vi "sensor count.vi"(0 "sensor thr array":dbl[](array[numeric]), 1 "debounce time":dbl=0.25 format="%#_13g", 5 "capture y or no ?":bool, 7 "sensor data":dbl[](array[numeric]), 9 "counter input":dbl, 11 "counting role":T1(ring), 12 "error in":errorcluster, 13 "falling level thr":dbl=59000.0 format="%#_13g") -> (2 "machine pallet stop":bool, 3 "column count":bool, 4 "capture trigger":bool, 6 "sensor counter":bool, 8 "speed":dbl, 10 "counter out":dbl, 14 "pallet detect":bool, 15 "error out":errorcluster)   [LabVIEW 2019]
uses:
  <vilib>/measure/mamon.llb/Trigger Detection for 1 Channel.vi
  <vilib>/measure/NI_MAPro.lvlib
panel:
  out "coloumn read time 2":dbl caption="Elapsed Time (s)"
  out "coloumn read time":dbl caption="Elapsed Time (s)"
  out "Numeric 3":i32=1
  out "Numeric 2":i32=1
  out "Numeric":i32=1
  out "Elapsed Time (s) 2":dbl caption="Elapsed Time (s)"
  out "Elapsed Time (s)":dbl
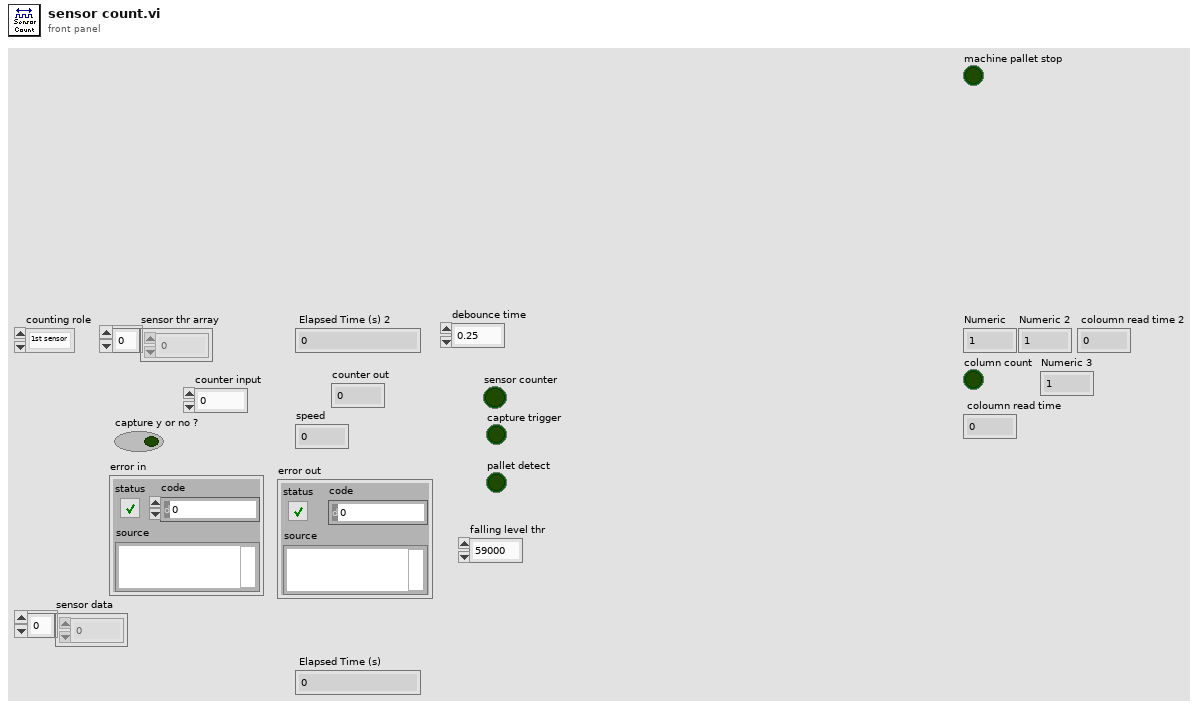
[diagram p1: front panel]
types:
  T1 = enum16{"1st sensor", "2nd sensor", "3rd sensor", "1st+2nd", "1st+3rd", "2nd+3rd", "1st+2nd+3rd"}
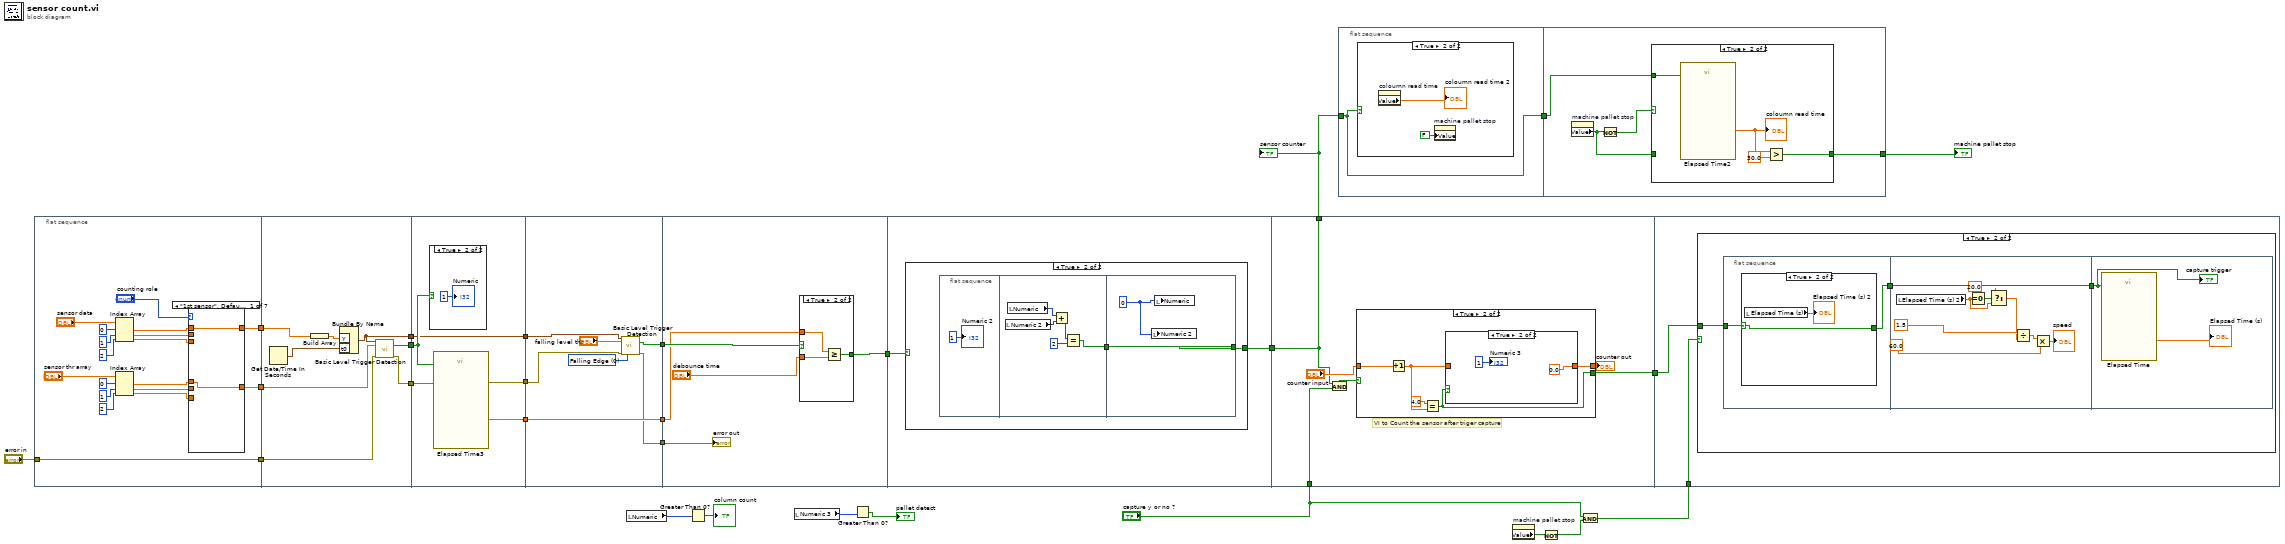
[diagram p0: block diagram]
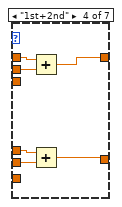
[diagram p4: hidden frame]
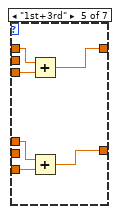
[diagram p5: hidden frame]
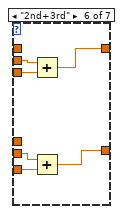
[diagram p6: hidden frame]
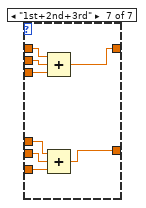
[diagram p7: hidden frame]
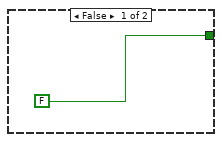
[diagram p10: hidden frame]
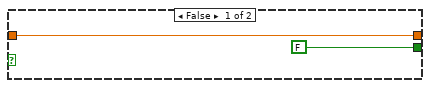
[diagram p11: hidden frame]
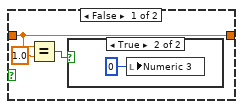
[diagram p12: hidden frame]
diagram:
  n1 = flat-sequence {
    tunnel: "error in" -> [w30]
    tunnel: [w30] -> w18
    tunnel: [w29] -> w17
    tunnel: [w28] -> w16
    tunnel: w18 -> [w85]
    tunnel: w17 -> [w84]
    tunnel: w16 -> [w83]
    tunnel: [w82] -> w15
    tunnel: [w81] -> w14
    tunnel: [w79] -> w12
    tunnel: w15 -> [w90]
    tunnel: w14 -> [w89]
    tunnel: [w88] -> w13
    tunnel: w12 -> [w88]
    tunnel: [w87] -> w11
    tunnel: [w86] -> w8
    tunnel: w13 -> [w96]
    tunnel: w11 -> [w95]
    tunnel: [w94] -> w10
    tunnel: [w93] -> w9
    tunnel: w8 -> [w93]
    tunnel: [w92] -> w1
    tunnel: w10 -> [w103]
    tunnel: w9 -> [w102]
    tunnel: [w101] -> w7
    tunnel: w1 -> [w100]
    tunnel: w7 -> [w109]
    tunnel: [w108] -> w6
    tunnel: w6 -> [w123]
    tunnel: [w123] -> w5
    tunnel: "capture y or no ?" -> [w122]
    tunnel: [w121] -> w4
    tunnel: w4 -> [w141]
    tunnel: w2 -> [w140]
    frame #0 {
      n2 = Index Array(array="sensor data", index #1=0 ("index"), index #2=1 ("index"), index #3=2 ("index")) -> (element #1=w43:dbl, element #2=w44:dbl, element #3=w45:dbl)
      n3 = Index Array(array="sensor thr array", index #1=0 ("index"), index #2=1 ("index"), index #3=2 ("index")) -> (element #1=w39:dbl, element #2=w40:dbl, element #3=w41:dbl)
      n4 = case shown="\"1st sensor\", Default" "counting role" {
        tunnel: w43 -> [w47 _ _ w55 w63 _ w77]
        tunnel: w39 -> [w46 _ _ w56 w61 _ w74]
        tunnel: w44 -> [_ w49 _ w57 _ w69 w76]
        tunnel: w45 -> [_ _ w51 _ w62 w68 w75]
        tunnel: w40 -> [_ w48 _ w54 _ w67 w73]
        tunnel: w41 -> [_ _ w50 _ w60 w66 w72]
        tunnel: [w47 w49 w51 w53 w59 w65 w71] -> w29
        tunnel: [w46 w48 w50 w52 w58 w64 w70] -> w28
        frame "1st sensor", Default {
        }
        frame "2nd sensor" {
        }
        frame "3rd sensor" {
        }
        frame "1st+2nd" {
          n5 = Add(x=w55, y=w57) -> (x+y=w53:dbl)
          n6 = Add(x=w56, y=w54) -> (x+y=w52:dbl)
        }
        frame "1st+3rd" {
          n7 = Add(x=w63, y=w62) -> (x+y=w59:dbl)
          n8 = Add(x=w61, y=w60) -> (x+y=w58:dbl)
        }
        frame "2nd+3rd" {
          n9 = Add(x=w69, y=w68) -> (x+y=w65:dbl)
          n10 = Add(x=w67, y=w66) -> (x+y=w64:dbl)
        }
        frame "1st+2nd+3rd" {
          n11 = Compound Arithmetic op=ADD(w77, w76, w75) -> (w71:dbl)
          n12 = Compound Arithmetic op=ADD(w74, w73, w72) -> (w70:dbl)
        }
      }
    }
    frame #1 {
      n13 = Get Date/Time In Seconds() -> (seconds since 1Jan1904=w78:timestamp)
      n14 = Build Array(w84) -> (w80:dbl[])
      n15 = Bundle By Name("Y"=w80, "t0"=w78) -> (w79:waveform(dbl))  [unwired: 1 in]
      n16 = call-poly <vilib>:"Basic Level Trigger Detection.vi"("signal in"=w79, "level"=w83, "error in (no error)"=w85) -> ("trigger detected?"=w82:bool, "error out"=w81:errorcluster)  [unwired: 10 in, 1 out]
    }
    frame #2 {
      n17 = case shown="True" w90 {
        frame False {
        }
        frame True {
          "Numeric" <- 1
        }
      }
      n18 = call "Elapsed Time3"("Reset"=w90, "error in (no error)"=w89) -> ("Elapsed Time (s)"=w86:dbl, "error out"=w87:errorcluster)  [unwired: 10 in, 6 out]
    }
    frame #3 {
      w97 = u16 0 items=["Falling Edge", "Rising Edge"] ("trigger slope")
      n19 = call-poly <vilib>:"Basic Level Trigger Detection.vi"("signal in"=w96, "level"="falling level thr", "error in (no error)"=w95, "trigger slope"=w97) -> ("trigger detected?"=w94:bool, "error out"=w92:errorcluster)  [unwired: 9 in, 1 out]
    }
    frame #4 {
      n20 = case shown="True" w103 {
        selector: w103 -> [w104 _]
        tunnel: w102 -> [_ w107]
        tunnel: [w104 w106] -> w101
        tunnel: "debounce time" -> [_ w105]
        frame False {
        }
        frame True {
          n21 = Greater Or Equal?(x=w107, y=w105) -> (x >= y?=w106:bool)
        }
      }
      "error out" <- w100
    }
    frame #5 {
      n22 = case shown="True" w109 {
        tunnel: [FALSE w112] -> w108
        frame False {
        }
        frame True {
          n23 = flat-sequence {
            tunnel: [w114] -> w111
            tunnel: [w120] -> w112
            tunnel: w111 -> [w120]
            frame #0 {
              "Numeric 2" <- 1
            }
            frame #1 {
              n24 = local read "Numeric 2"() -> (w117:i32)
              n25 = local read "Numeric"() -> (w118:i32)
              n26 = Add(x=w118, y=w117) -> (x+y=w116:i32)
              n27 = Equal?(x=w116, y=2) -> (x = y?=w114:bool)
            }
            frame #2 {
              w119 = 0 ("Numeric")
              n28 = local write "Numeric 2"(w119) -> ()
              n29 = local write "Numeric"(w119) -> ()
            }
          }
        }
      }
    }
    frame #6 {
      # "VI to Count the sensor after triger capture"
      n30 = And(x=w123, y=w122) -> (x .and. y?=w126:bool)
      n31 = case shown="True" w126 {
        tunnel: "counter input" -> [w128 w132]
        tunnel: [w128 w130] -> w124
        tunnel: [FALSE w129] -> w121
        frame False {
        }
        frame True {
          n32 = Increment(x=w132) -> (x+1=w131:dbl)
          n33 = Equal?(x=4.0, y=w131) -> (x = y?=w129:bool)
          n34 = case shown="True" w129 {
            tunnel: w131 -> [w136 _]
            tunnel: [w136 0.0 ("counter out")] -> w130
            frame False {
              n35 = Equal?(x=w136, y=1.0) -> (x = y?=w134:bool)
              n36 = case shown="True" w134 {
                frame False {
                }
                frame True {
                  n37 = local write "Numeric 3"(0 ("Numeric 3")) -> ()
                }
              }
            }
            frame True {
              "Numeric 3" <- 1
            }
          }
        }
      }
      "counter out" <- w124
    }
    frame #7 {
      n38 = case shown="True" w140 {
        tunnel: w141 -> [_ w144]
        frame False {
        }
        frame True {
          n39 = flat-sequence {
            tunnel: w144 -> [w146]
            tunnel: [w145] -> w143
            tunnel: w143 -> [w158]
            tunnel: [w158] -> w142
            tunnel: w142 -> [w159]
            frame #0 {
              n40 = case shown="True" w146 {
                selector: w146 -> [w147 w149]
                tunnel: [w147 w149] -> w145
                frame False {
                }
                frame True {
                  n41 = local read "Elapsed Time (s)"() -> (→"Elapsed Time (s) 2":dbl)
                }
              }
            }
            frame #1 {
              n42 = local read "Elapsed Time (s) 2"() -> (w151:dbl)
              n43 = Equal To 0?(x=w151) -> (x = 0?=w153:bool)
              n44 = Select(t=20.0, s=w153, f=w151) -> (s? t:f=w150:dbl)
              n45 = Divide(x=1.5, y=w150) -> (x/y=w156:dbl)
              n46 = Multiply(x=w156, y=60.0) -> (x*y=→"speed":dbl)
            }
            frame #2 {
              n47 = call "Elapsed Time"("Reset"=w159) -> ("Elapsed Time (s)"=→"Elapsed Time (s)":dbl)  [unwired: 11 in, 7 out]
              "capture trigger" <- w159
            }
          }
        }
      }
    }
  }
  n48 = local read "Numeric"() -> (w27:i32)
  n49 = Greater Than 0?(x=w27) -> (x > 0?=→"column count":bool)
  n50 = local read "Numeric 3"() -> (w25:i32)
  n51 = Greater Than 0?(x=w25) -> (x > 0?=→"pallet detect":bool)
  n52 = flat-sequence {
    tunnel: w5 -> [w161]
    tunnel: [w161] -> w23
    tunnel: w23 -> [w167]
    tunnel: [w165] -> w20
    frame #0 {
      n53 = case shown="True" w161 {
        frame False {
        }
        frame True {
          n54 = property on="coloumn read time" class="DigNum (strict)"() -> ("Value"=→"coloumn read time 2":dbl)  [unwired: 2 in, 2 out]
          n55 = property on="machine pallet stop" class="Bool (strict)"("Value"=FALSE ("machine pallet stop")) -> ()  [unwired: 2 in, 2 out]
        }
      }
    }
    frame #1 {
      n56 = property on="machine pallet stop" class="Bool (strict)"() -> ("Value"=w164:bool)  [unwired: 2 in, 2 out]
      n57 = Not(x=w164) -> (.not. x?=w166:bool)
      n58 = case shown="True" w166 {
        tunnel: w167 -> [_ w172]
        tunnel: [w168 w169] -> w165
        tunnel: w164 -> [w168 _]
        frame False {
        }
        frame True {
          n59 = call "Elapsed Time2"("Reset"=w172) -> ("Elapsed Time (s)"=w171:dbl)  [unwired: 11 in, 7 out]
          "coloumn read time" <- w171
          n60 = Greater?(x=w171, y=30.0) -> (0:w169:bool)
        }
      }
    }
  }
  n61 = property on="machine pallet stop" class="Bool (strict)"() -> ("Value"=w22:bool)  [unwired: 2 in, 2 out]
  n62 = Not(x=w22) -> (.not. x?=w21:bool)
  n63 = And(x="capture y or no ?", y=w21) -> (x .and. y?=w2:bool)
  "machine pallet stop" <- w20
  "sensor counter" <- w5
